vi "WAIT_FOR_CAMERA.vi"(10 "argv":string[](array[string]), 11 "args":u8) -> ()   [LabVIEW 2011]
uses:
  <vilib>/Rock Robotics/WPI/DriverStation/WPI_DriverStationStatusErrorCache.ctl
  Auto_Conf.vi
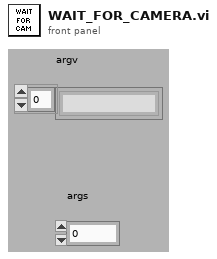
[diagram p1: front panel]
types:
  T1 = typedef "WPI_DriverStationStatusErrorCache.ctl" = enum16{"Get", "Set"}
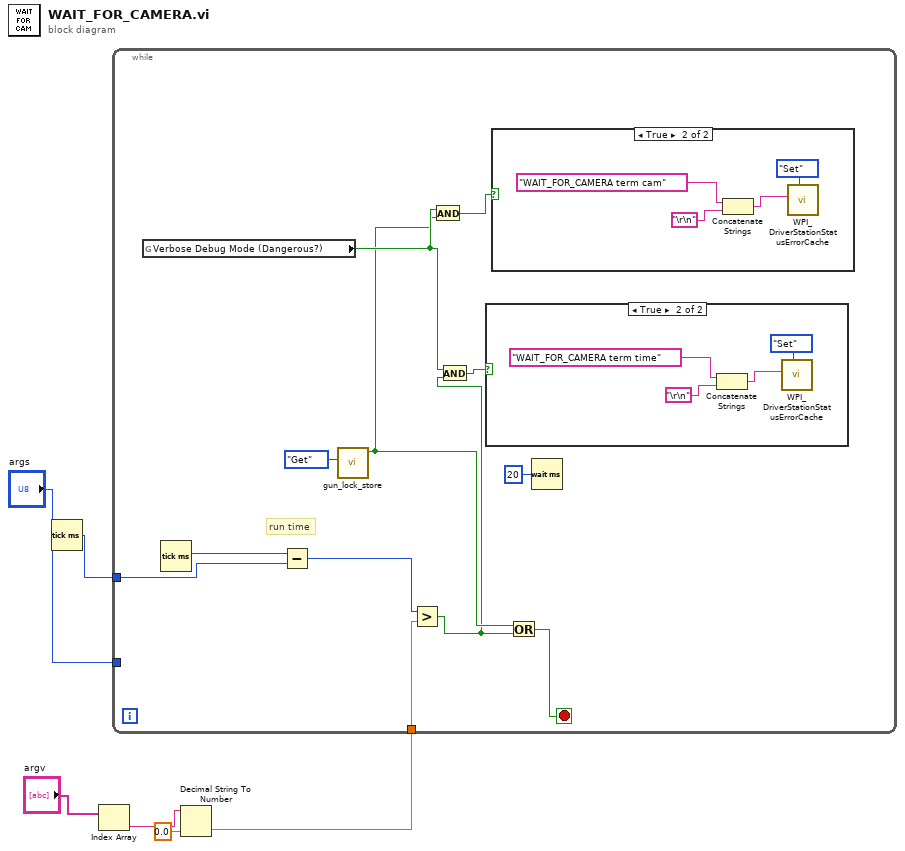
[diagram p0: block diagram]
diagram:
  n1 = Tick Count (ms)() -> (millisecond timer value=w1:u32)
  n2 = Index Array(array="argv") -> (element=w4:string)  [unwired: 1 in]
  n3 = Decimal String To Number(string=w4, default (0L)=0.0 ("default (0 I32)")) -> (number=w2:dbl)  [unwired: 1 in, 1 out]
  n4 = while {
    tunnel: "args" -> [_]
    tunnel: w2 -> [w16]
    tunnel: w1 -> [w9]
    stop <- w15 stop-if-true
    # "run time"
    n5 = global read "Auto_Conf.vi" "Verbose Debug Mode (Dangerous?)"() -> (w11:bool)
    n6 = Tick Count (ms)() -> (millisecond timer value=w17:u32)
    n7 = Subtract(x=w17, y=w9) -> (x-y=w8:u32)
    n8 = call "gun_lock_store.vi"("data_store_mode"=enum16{"Set", "Get"}."Get") -> ("Lock"=w10:bool)  [unwired: 10 in]
    n9 = Greater?(x=w8, y=w16) -> (0:w7:bool)
    n10 = And(x=w11, y=w10) -> (x .and. y?=w13:bool)
    n11 = And(x=w11, y=w7) -> (x .and. y?=w12:bool)
    n12 = case shown="True" w12 {
      frame False {
      }
      frame True {
        n13 = Concatenate Strings("WAIT_FOR_CAMERA term time" ("string"), "\r\n") -> (w25:string)
        n14 = call <vilib>:"WPI_DriverStationStatusErrorCache.vi"("StatusErrorCacheOp"=WPI_DriverStationStatusErrorCache."Set", "Error String"=w25) -> ()  [unwired: 10 out]
      }
    }
    n15 = case shown="True" w13 {
      frame False {
      }
      frame True {
        n16 = Concatenate Strings("WAIT_FOR_CAMERA term cam" ("string"), "\r\n") -> (w21:string)
        n17 = call <vilib>:"WPI_DriverStationStatusErrorCache.vi"("StatusErrorCacheOp"=WPI_DriverStationStatusErrorCache."Set", "Error String"=w21) -> ()  [unwired: 10 out]
      }
    }
    n18 = Or(x=w10, y=w7) -> (x .or. y?=w15:bool)
    n19 = Wait (ms)(milliseconds to wait=u32 20) -> ()  [unwired: 1 out]
  }
